vi "LVClass_WavefrontCorrector Init.vi"(0 "WavefrontCorrector in":refnum<class "WavefrontCorrector.lvclass">, 5 "set_init_state_from_config_file":bool, 11 "error in (no error)":errorcluster) -> (4 "WavefrontCorrector out":refnum<class "WavefrontCorrector.lvclass">, 15 "error out":errorcluster)   [LabVIEW 2020, in "WavefrontCorrector.lvclass"]
doc: "Wavefront corrector parameter getter for parameter of type boolean.\n\n--------------------------------------------------------------------------------\n\n<B>correctorIn </B> : WavefrontCorrector object.\n<B>correctorOut </B> : WavefrontCorrector object.\n<B>parameter_name </B> : Name of the parameter.\n<B>value </B> : Value of the parameter.\n<B>ErrorIn </B> : Error\n<B>ErrorOut </B> : Error\n\n--------------------------------------------------------------------------------"
uses:
  WavefrontCorrector.lvclass
  WavefrontCorrector.lvclass/WavefrontCorrector.ctl
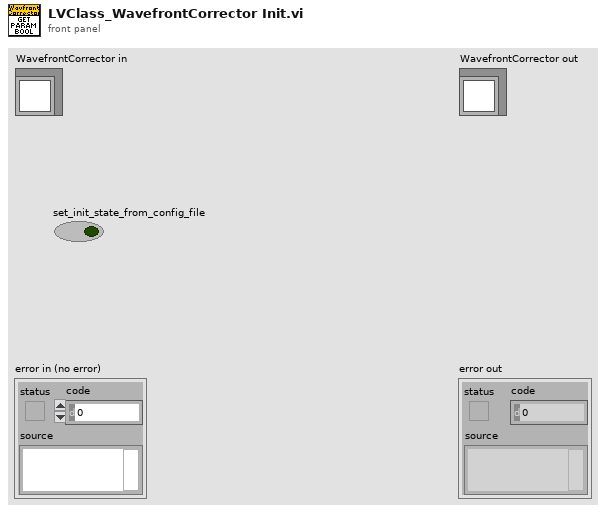
[diagram p1: front panel]
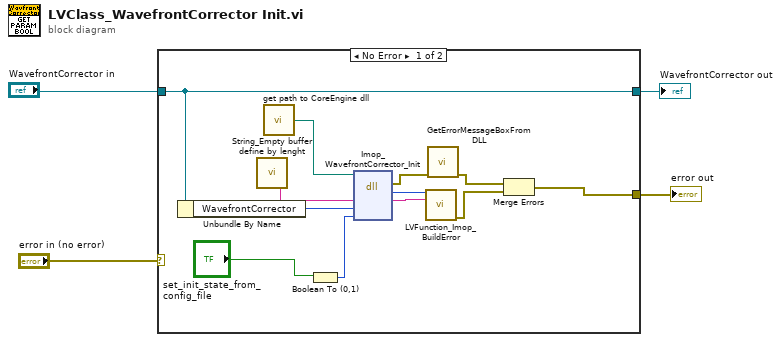
[diagram p0: block diagram]
diagram:
  n1 = case shown="No Error" "error in (no error)" {
    selector: "error in (no error)" -> [_ w18]
    tunnel: [w6 w18] -> w2
    tunnel: [w13 w17] -> w1
    tunnel: "WavefrontCorrector in" -> [w13 w17]
    frame No Error {
      n2 = Unbundle By Name(w13) -> ("WavefrontCorrector"=w14:i32)
      n3 = call "String_Empty buffer define by lenght.vi"() -> ("Empty buffer"=w10:string)  [unwired: 1 in]
      n4 = call "get path to CoreEngine dll.vi"() -> ("path to c_interface_vc100.dll"=w12:path)  [unwired: 12 in, 3 out]
      n5 = Boolean To (0,1)(Boolean="set_init_state_from_config_file") -> (0, 1=w9:i16)
      n6 = dll-call lib="D:/SOFTware/CoreEngine4_Suite/SVN_trunk/LV2011_interface/DLLs/c_interface_vc100.dll" fn="Imop_WavefrontCorrector_Init"(path in=w12, "message"=w10, "camera"=w14, "set_init_state_from_config_file"=w9) -> (error out=w11:errorcluster, "return type"=w16:i32, "message"=w15:string)  [unwired: 4 in, 1 out]
      n7 = call "LVFunction_Imop_BuildError.vi"("code"=w16, "String to Prepend to source (\"\")"=w15) -> ("error out"=w7:errorcluster)  [unwired: 13 in]
      n8 = call "GetErrorMessageBoxFromDLL.vi"("error IN"=w11) -> ("error OUT"=w8:errorcluster)  [unwired: 10 in]
      n9 = Merge Errors(w8, w7) -> (w6:errorcluster)
    }
    frame Error {
    }
  }
  "error out" <- w2
  "WavefrontCorrector out" <- w1
